vi "File_data_cinetica.vi"(8 "path in":path=path "C:/H2_Painel/painel_auto/00100_cinetica.txt", 9 "Nota 01":string, 10 "Sample name":string, 11 "File name":string) -> (0 "path":path)   [LabVIEW 2011]
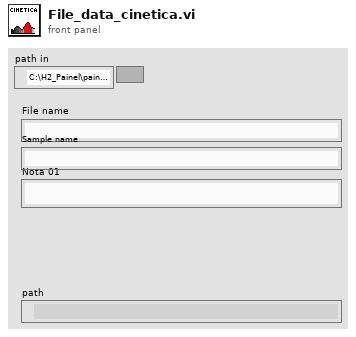
[diagram p1: front panel]
types:
  T1 = enum16{"open", "replace", "create", "open or create", "replace or create", "replace or create with confirmation"}
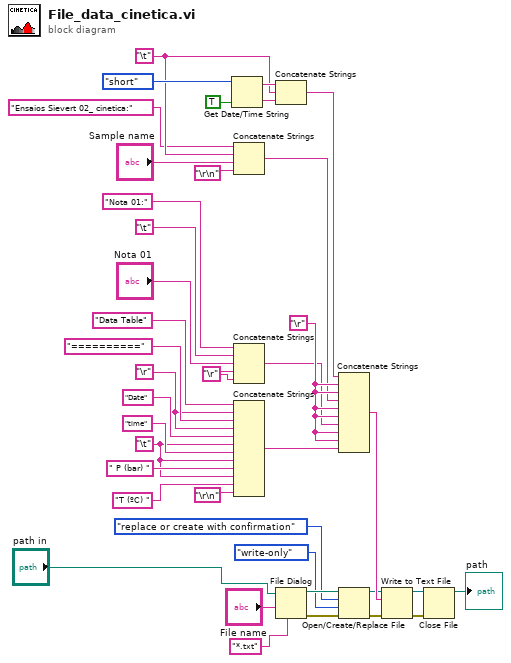
[diagram p0: block diagram]
diagram:
  w5 = "\t"
  w4 = "\r"
  w26 = "\r"
  w23 = "\r"
  w8 = "\t"
  n1 = Get Date/Time String(date format (0)=enum16{"short", "long", "abbreviated"}."short", want seconds? (F)=TRUE) -> (date string=w35:string, time string=w34:string)  [unwired: 1 in]
  n2 = Concatenate Strings("Ensaios Sievert 02_ cinetica:" ("string"), w8, "Sample name", "\r\n") -> (w6:string)
  n3 = Concatenate Strings("Nota 01:" ("Nota 4"), "\t", "Nota 01", w4, w4) -> (w21:string)
  n4 = Concatenate Strings("Data Table" ("string"), w26, "==========" ("string"), w26, "Date" ("string"), w5, "time" ("string"), w5, " P (bar) " ("string"), w5, "T (ºC) " ("string"), "\r\n") -> (w24:string)
  n5 = Concatenate Strings(w35, w8, w34) -> (w25:string)
  n6 = File Dialog(6:"*.txt" ("pattern label"), 9:"File name", 11:"path in") -> (0:w19:errorcluster, 3:w20:path)  [unwired: 2 in, 4 out]
  n7 = Concatenate Strings(w25, w23, w23, w6, w23, w23, w21, w23, w23, w24) -> (w33:string)
  n8 = Open/Create/Replace File(file path (use dialog)=w20, error in=w19, operation (0:open)=T1."replace or create with confirmation", access (0:read/write)=enum16{"read/write", "read-only", "write-only"}."write-only") -> (refnum out=w16:refnum<file>, error out=w15:errorcluster)  [unwired: 3 out]
  n9 = Write to Text File(file (use dialog)=w16, text=w33, error in=w15) -> (refnum out=w14:refnum<file>, error out=w11:errorcluster)  [unwired: 1 in, 1 out]
  n10 = Close File(refnum=w14, error in=w11) -> (path=→"path":path)  [unwired: 1 out]
